vi "SetTurretOutput.vi"(9 "Use PID?":bool, 10 "Turret Setpoint Angles":dbl[](array[numeric]), 11 "All Pods In":T17(array[cluster])) -> (2 "Motor Outputs":dbl[](array[numeric]), 3 "All Pods out":T17(array[cluster]))   [LabVIEW 2014]
uses:
  <vilib>/Rock Robotics/WPI/MotorControl/WPI_MotorControlDeviceRef.ctl
  <vilib>/Rock Robotics/WPI/MotorControl/WPI_MotorControlType.ctl
  <vilib>/Rock Robotics/SystemInterfaces/Typedef/FPGA_TypedefDigitalModule.ctl
  <vilib>/Rock Robotics/SystemInterfaces/DIO/FPGA_DIOPWMChannel.ctl
  <vilib>/Rock Robotics/WPI/PWM/WPI_PWMDeadband.ctl
  <vilib>/Rock Robotics/WPI/CAN/Jaguar/SubVIs/WPI_CANJaguar_ControlMode.ctl
  <vilib>/Rock Robotics/WPI/CAN/TalonSRX/WPI_CANTalonSRX_APIControlMode.ctl
  <vilib>/Rock Robotics/WPI/PWM/WPI_PWMTransform_ConPane.ctl
  <vilib>/Rock Robotics/WPI/AnalogChannel/WPI_AnalogChannelDevRef.ctl
  <vilib>/Rock Robotics/SystemInterfaces/Typedef/FPGA_TypedefAnalogModule.ctl
  <vilib>/Rock Robotics/SystemInterfaces/AI/FPGA_AIChannel.ctl
  <vilib>/Rock Robotics/WPI/Encoder/WPI_EncoderDevRef.ctl
  <vilib>/Rock Robotics/SystemInterfaces/Encoder/FPGA_EncoderIdx.ctl
  <vilib>/Rock Robotics/SystemInterfaces/Counter/FPGA_CounterCtrSystemIndex.ctl
  <vilib>/Rock Robotics/WPI/Encoder/WPI_EncoderType.ctl
  Variables/Physical data.vi
  <vilib>/addons/control/pid/pid.llb/PID (DBL Array).vi
  <vilib>/addons/control/pid/NI_PID_pid.lvlib
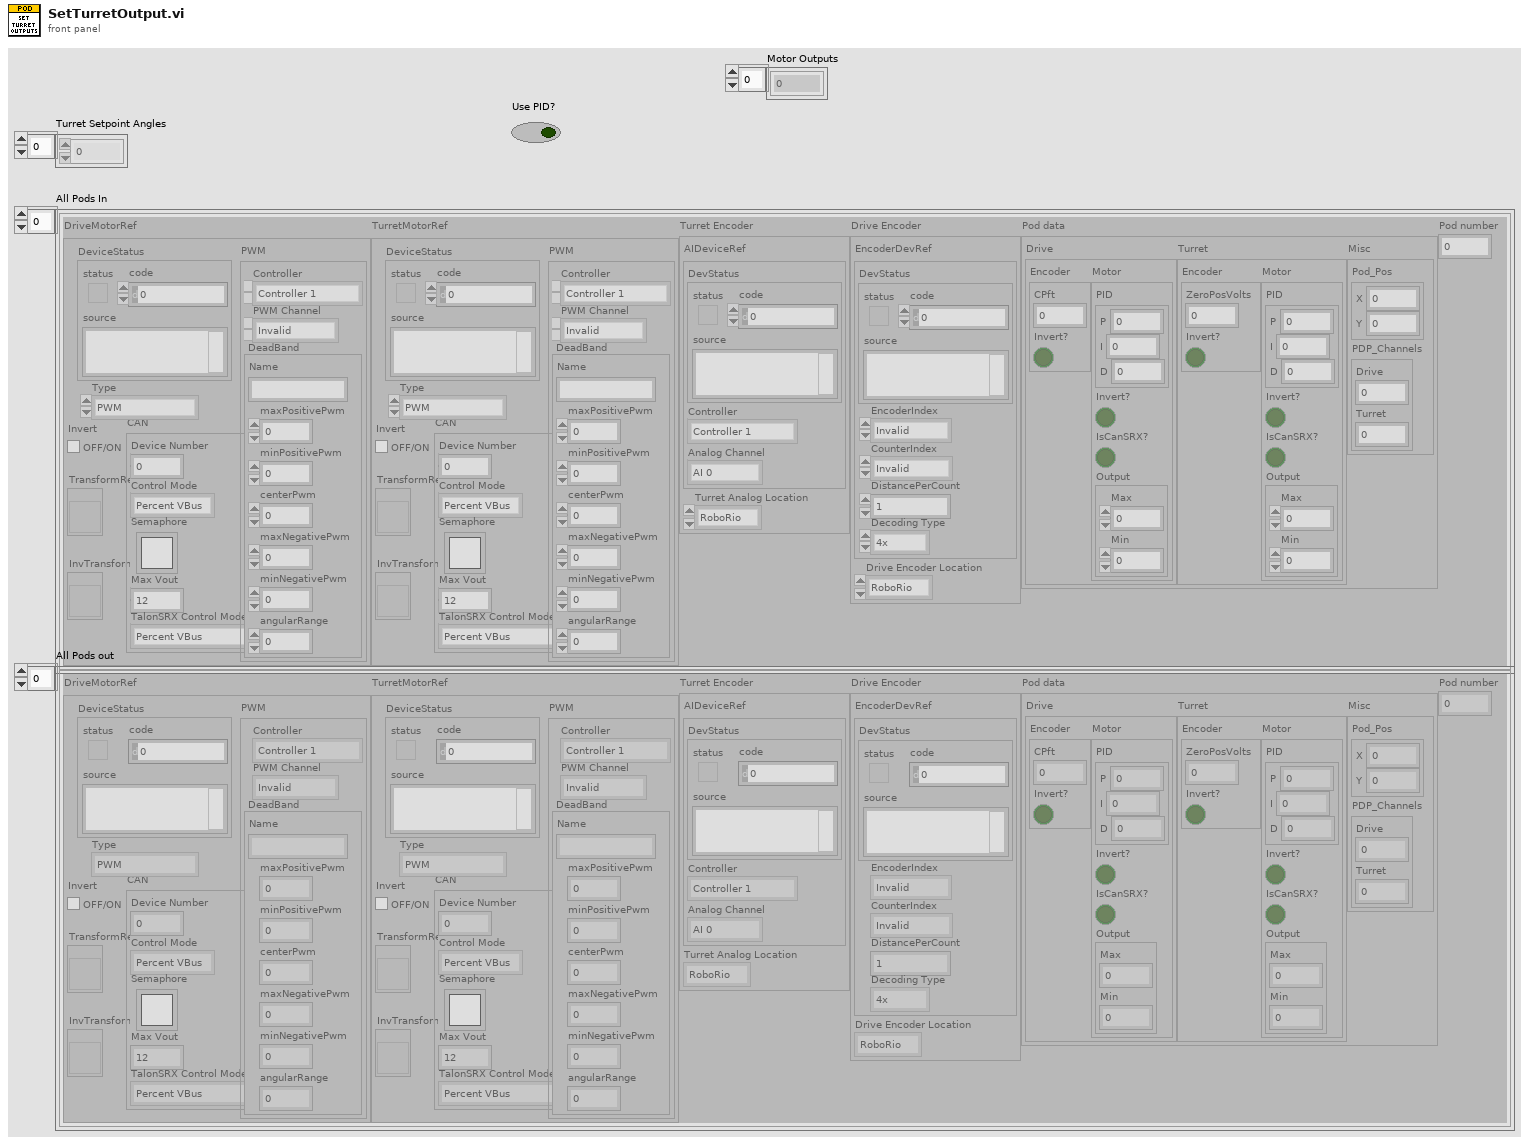
[diagram p1: front panel]
types:
  T1 = typedef "WPI_MotorControlDeviceRef.ctl" = cluster{"DeviceStatus":errorcluster, "Type":T2, "PWM":cluster{"Controller":T3, "PWM Channel":T4, "DeadBand":T5}, "CAN":cluster{"Device Number":u8, "Control Mode":T6, "Semaphore":T7, "Max Vout":dbl, "TalonSRX Control Mode":T8}, "Invert":bool, "TransformRef":T9, "InvTransformRef":T9}
  T2 = typedef "WPI_MotorControlType.ctl" = enum16{"PWM", "CAN", "CANTalonSRX"}
  T3 = typedef "FPGA_TypedefDigitalModule.ctl" = enum16{"Controller 1"}
  T4 = typedef "FPGA_DIOPWMChannel.ctl" = enum8{"PWM 0", "PWM 1", "PWM 2", "PWM 3", "PWM 4", "PWM 5", "PWM 6", "PWM 7", "PWM 8", "PWM 9", "PWM MXP 0", "PWM MXP 1", "PWM MXP 2", "PWM MXP 3", "PWM MXP 4", "PWM MXP 5", "PWM MXP 6", "PWM MXP 7", "PWM MXP 8", "PWM MXP 9", "Invalid"}
  T5 = typedef "WPI_PWMDeadband.ctl" = cluster{"Name":string, "maxPositivePwm":i32, "minPositivePwm":i32, "centerPwm":i32, "maxNegativePwm":i32, "minNegativePwm":i32, "angularRange":u16}
  T6 = typedef "WPI_CANJaguar_ControlMode.ctl" = enum8{"Percent VBus", "Current", "Speed", "Position", "Voltage"}
  T7 = typedef "Semaphore RefNum" = refnum<k1>
  T8 = typedef "WPI_CANTalonSRX_APIControlMode.ctl" = enum8{"Percent VBus", "Speed", "Position", "Slave", "Unchanged / Invalid"}
  T9 = typedef "WPI_PWMTransform_ConPane.ctl" = refnum<vi>
  T10 = typedef "WPI_AnalogChannelDevRef.ctl" = cluster{"DevStatus":errorcluster, "Controller":T11, "Analog Channel":T12}
  T11 = typedef "FPGA_TypedefAnalogModule.ctl" = enum16{"Controller 1"}
  T12 = typedef "FPGA_AIChannel.ctl" = enum8{"AI 0", "AI 1", "AI 2", "AI 3", "AI MXP 0", "AI MXP 1", "AI MXP 2", "AI MXP 3", "Invalid"}
  T13 = typedef "WPI_EncoderDevRef.ctl" = cluster{"DevStatus":errorcluster, "EncoderIndex":T14, "CounterIndex":T15, "DistancePerCount":dbl, "Decoding Type":T16}
  T14 = typedef "FPGA_EncoderIdx.ctl" = enum8{"Enc 0", "Enc 1", "Enc 2", "Enc 3", "Enc 4", "Enc 5", "Enc 6", "Enc 7", "Invalid"}
  T15 = typedef "FPGA_CounterCtrSystemIndex.ctl" = enum8{"Ctr 0", "Ctr 1", "Ctr 2", "Ctr 3", "Ctr 4", "Ctr 5", "Ctr 6", "Ctr 7", "Invalid"}
  T16 = typedef "WPI_EncoderType.ctl" = enum16{"1x", "2x", "4x"}
  T17 = cluster{"DriveMotorRef":T1, "TurretMotorRef":T1, "Turret Encoder":cluster{"AIDeviceRef":T10, "Turret Analog Location":enum16{"RoboRio", "Drive SRX", "Turret SRX"}}, "Drive Encoder":cluster{"EncoderDevRef":T13, "Drive Encoder Location":enum16{"RoboRio", "Drive SRX", "Turret SRX"}}, "Pod data":cluster{"Drive":cluster{"Encoder":cluster{"CPft":dbl, "Invert?":bool}, "Motor":cluster{"PID":cluster{"P":dbl, "I":dbl, "D":dbl}, "Invert?":bool, "IsCanSRX?":bool, "Output":cluster{"Max":dbl, "Min":dbl}}}, "Turret":cluster{"Encoder":cluster{"ZeroPosVolts":dbl, "Invert?":bool}, "Motor":cluster{"PID":cluster{"P":dbl, "I":dbl, "D":dbl}, "Invert?":bool, "IsCanSRX?":bool, "Output":cluster{"Max":dbl, "Min":dbl}}}, "Misc":cluster{"Pod_Pos":cluster{"X":dbl, "Y":dbl}, "PDP_Channels":cluster{"Drive":i32, "Turret":i32}}}, "Pod number":i32}[]
  T18 = typedef "NI_Matrix.lvlib/RealMatrix.ctl" = dbl[][]
  T19 = cluster{"All Pod State Data":cluster{"Drive":cluster{"Drive Motor Output":dbl, "Wheel RPM":dbl, "Linear speed":dbl, "Linear acceleration":dbl, "Encoder Output":dbl, "Vmot":dbl, "Imot":dbl, "Torque":dbl, "Angular Momentum":dbl}, "Turret":cluster{"Turret Motor Output":dbl, "Turret Angle":dbl, "Turret velocity":dbl, "Turret acceleration":dbl, "Encoder Output":dbl, "Vmot":dbl, "Imot":dbl, "Torque":dbl, "Angular Momentum":dbl}, "Pod position (RCS)":cluster{"X":dbl, "Y":dbl, "Z":dbl}}[], "Global Robot Data":cluster{"Position Data":cluster{"Robot Position":cluster{"X":dbl, "Y":dbl, "Z":dbl}, "Robot Velocity":cluster{"X":dbl, "Y":dbl, "Z":dbl}, "Robot Acceleration":cluster{"X":dbl, "Y":dbl, "Z":dbl}}, "Rotation Data":cluster{"Angular Position":cluster{"X":dbl, "Y":dbl, "Z":dbl}, "Angular Velocity":cluster{"X":dbl, "Y":dbl, "Z":dbl}, "Angular Acceleration":cluster{"X":dbl, "Y":dbl, "Z":dbl}}}, "Inertial Characteristics":cluster{"Center of Mass (RCS)":cluster{"X":dbl, "Y":dbl, "Z":dbl}, "Mass Elements":cluster{"X":dbl, "Y":dbl, "Z":dbl, "Mass":dbl, "Name":string}[], "Center of Rotation (RCS)":cluster{"X":dbl, "Y":dbl, "Z":dbl}, "Tensor of Inertia":T18}}
  T20 = cluster{"Drive":cluster{"Drive Motor Output":dbl, "Wheel RPM":dbl, "Linear speed":dbl, "Linear acceleration":dbl, "Encoder Output":dbl, "Vmot":dbl, "Imot":dbl, "Torque":dbl, "Angular Momentum":dbl}, "Turret":cluster{"Turret Motor Output":dbl, "Turret Angle":dbl, "Turret velocity":dbl, "Turret acceleration":dbl, "Encoder Output":dbl, "Vmot":dbl, "Imot":dbl, "Torque":dbl, "Angular Momentum":dbl}, "Pod position (RCS)":cluster{"X":dbl, "Y":dbl, "Z":dbl}}[]
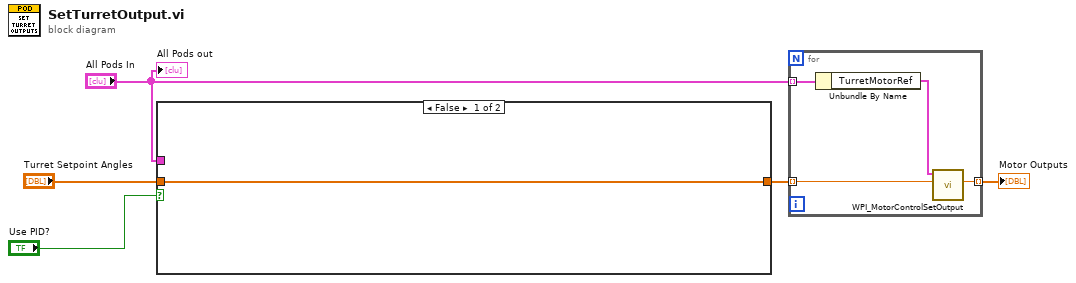
[diagram p0: block diagram]
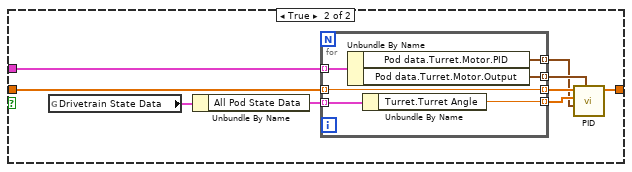
[diagram p2: hidden frame]
diagram:
  n1 = case shown="False" "Use PID?" {
    tunnel: "Turret Setpoint Angles" -> [w6 w15]
    tunnel: "All Pods In" -> [_ w8]
    tunnel: [w6 w7] -> w3
    frame False {
    }
    frame True {
      n2 = global read "Physical data.vi" "Drivetrain State Data"() -> (w14:T19)
      n3 = Unbundle By Name(w14) -> ("All Pod State Data"=w13:T20)
      n4 = for {
        tunnel: w15 -> [w16] mode=indexing
        tunnel: w8 -> [w21] mode=indexing
        tunnel: w13 -> [w20] mode=indexing
        tunnel: [w19] -> w9 mode=indexing
        tunnel: [w18] -> w10 mode=indexing
        tunnel: [w17] -> w12 mode=indexing
        tunnel: [w16] -> w11 mode=indexing
        n5 = Unbundle By Name(w21) -> ("Pod data.Turret.Motor.PID"=w19:cluster{"P":dbl, "I":dbl, "D":dbl}, "Pod data.Turret.Motor.Output"=w17:cluster{"Max":dbl, "Min":dbl})
        n6 = Unbundle By Name(w20) -> ("Turret.Turret Angle"=w18:dbl)
      }
      n7 = call-poly <vilib>:"PID.vi"("output range"=w12, "PID gains"=w9, "process variable"=w10, "setpoint"=w11) -> ("output"=w7:dbl[])  [unwired: 6 in, 1 out]
    }
  }
  n8 = for {
    tunnel: "All Pods In" -> [w25] mode=indexing
    tunnel: w3 -> [w23] mode=indexing
    tunnel: [w22] -> w2 mode=indexing
    n9 = Unbundle By Name(w25) -> ("TurretMotorRef"=w24:T1)
    n10 = call <vilib>:"WPI_MotorControlSetOutput.vi"("Output"=w23, "MotorControlDevRef"=w24) -> ("Motor Output"=w22:dbl)  [unwired: 7 in, 2 out]
  }
  "Motor Outputs" <- w2
  "All Pods out" <- "All Pods In"
